vi "RH_Auto.vi"() -> ()   [LabVIEW 2012]
uses:
  <vilib>/ptbypt/NI_PtbyPt.lvlib
panel:
  out "Resistance [Ohm]":dbl=29.242166666666666 format="%#_6f"
  out "Lockin y (V)":dbl=2.45572e-05
  out "Lockin x (V)":dbl=0.000873212
  in  "On:Delta\nOff:Lock-in":bool
  in  "I for Lockin [A]":dbl=3e-05 format="%#_6e"
  out "Lockin Y (V)":dbl=2.41996e-05
  out "Lockin X (V)":dbl=0.000877265
  in  "Lockin SR830":refnum<visa-resource-name>="GPIB1::8::INSTR"
  in  "T-ramp off":bool
  in  "Main sorb T control":bool
  in  "Wait [min]":i32
  in  "LakeShore335":refnum<visa-resource-name>="COM4"
  in  "Temp control off":bool
  out "temp [K]":dbl=10.052
  out "Waiting T-stability":bool caption="stabilizing"
  in  "Set Initial Field":bool
  in  "Field [T]":dbl
  in  "Period [s]":dbl=0.5 caption="Delay Time (s)"
  in  "Measure R-T":bool
  in  "Save R-T":bool
  out "R-T":cluster{"X":dbl[], "Y":dbl[]}[](graph) caption="XY Graph"
  out "Rate [K/min]":dbl=-0.3439169609352251 format="%#_6f"
  in  "Reset":bool
  in  "Stop":bool
  in  "Pause off":bool
  in  "Compliance [V]":dbl=0.5 format="%#_6f"
  out "R-H":cluster{"X":dbl[], "Y":dbl[]}[](graph) caption="XY Graph"
  in  "Reset":bool
  in  "Folder":path=path "C:/User Data/Bart" caption="Filename"
  out "Filename Out":path=path "C:/User Data/Bart/CG013_RH_2_10.00K"
  in  "File name":string="CG013_RH_2"
  out "VTI [K]":dbl=9.9728
  out "VTI [K]":dbl=9.8121
  out "Sample Temp [K]":dbl=10.114
  out "Magnetic Field [T]":dbl=-2.97563
  out "Delta reading [Ohm]":dbl
  out "Delta Reading [Ohm]":dbl=11.9426813
  out "Sample Temp [K]":dbl=10.057
  in  "Abort Delta":bool
  in  "Arm Delta":bool
  in  "DELAY [sec]":dbl=0.002 format="%#_6e"
  in  "I-HIGH [A]":dbl=1e-06 format="%#_6e"
  in  "Measure R-H":bool
  in  "Rate [K/min]":dbl=0.5
  in  "Set Temp [K]":dbl=1.0
  in  "Set Temperature":bool
  out "Magnetic Field [T]":dbl=-2.94426
  in  "Rate [T/min]":dbl=0.5
  in  "Set Field [T]":dbl=3.0
  in  "Set Field":bool
  in  "Keithley":refnum<visa-resource-name>="GPIB1::20::INSTR"
  in  "Skip":bool
  in  "Wait T-stable [min]":i32=10
  in  "period (s)":dbl=0.5 min=0.0 max=1111.0 step=0.1
  in  "stop 2":bool caption="Pause"
  in  "Wait field stable [sec]":dbl=20.0
  in  "Magnet Power supply":refnum<visa-resource-name>="COM7"
  in  "Set Field [T]   Rate [T/min]":dbl[][](array[numeric])=[[0.0, 0.5], [3.0, 0.5], [0.0, 0.5], [-3.0, 0.5]]
  in  "Set Temp [K]  Rate [K/min]":dbl[][](array[numeric])=[[10.0, 3.0]]
  in  "LakeShore340":refnum<visa-resource-name>="GPIB1::4::INSTR"
  out "error out 3":errorcluster={"status"=FALSE, "code"=1073676294, "source"="VISA Read in RH_Auto.vi"}
  out "error out 2":errorcluster={"status"=FALSE, "code"=1073676294, "source"="VISA Read in RH_Auto.vi"}
  out "error out":errorcluster={"status"=FALSE, "code"=1073676294, "source"="VISA Read in RH_Auto.vi"}
  # "Manual control"
  # "R-H Auto Measurement"
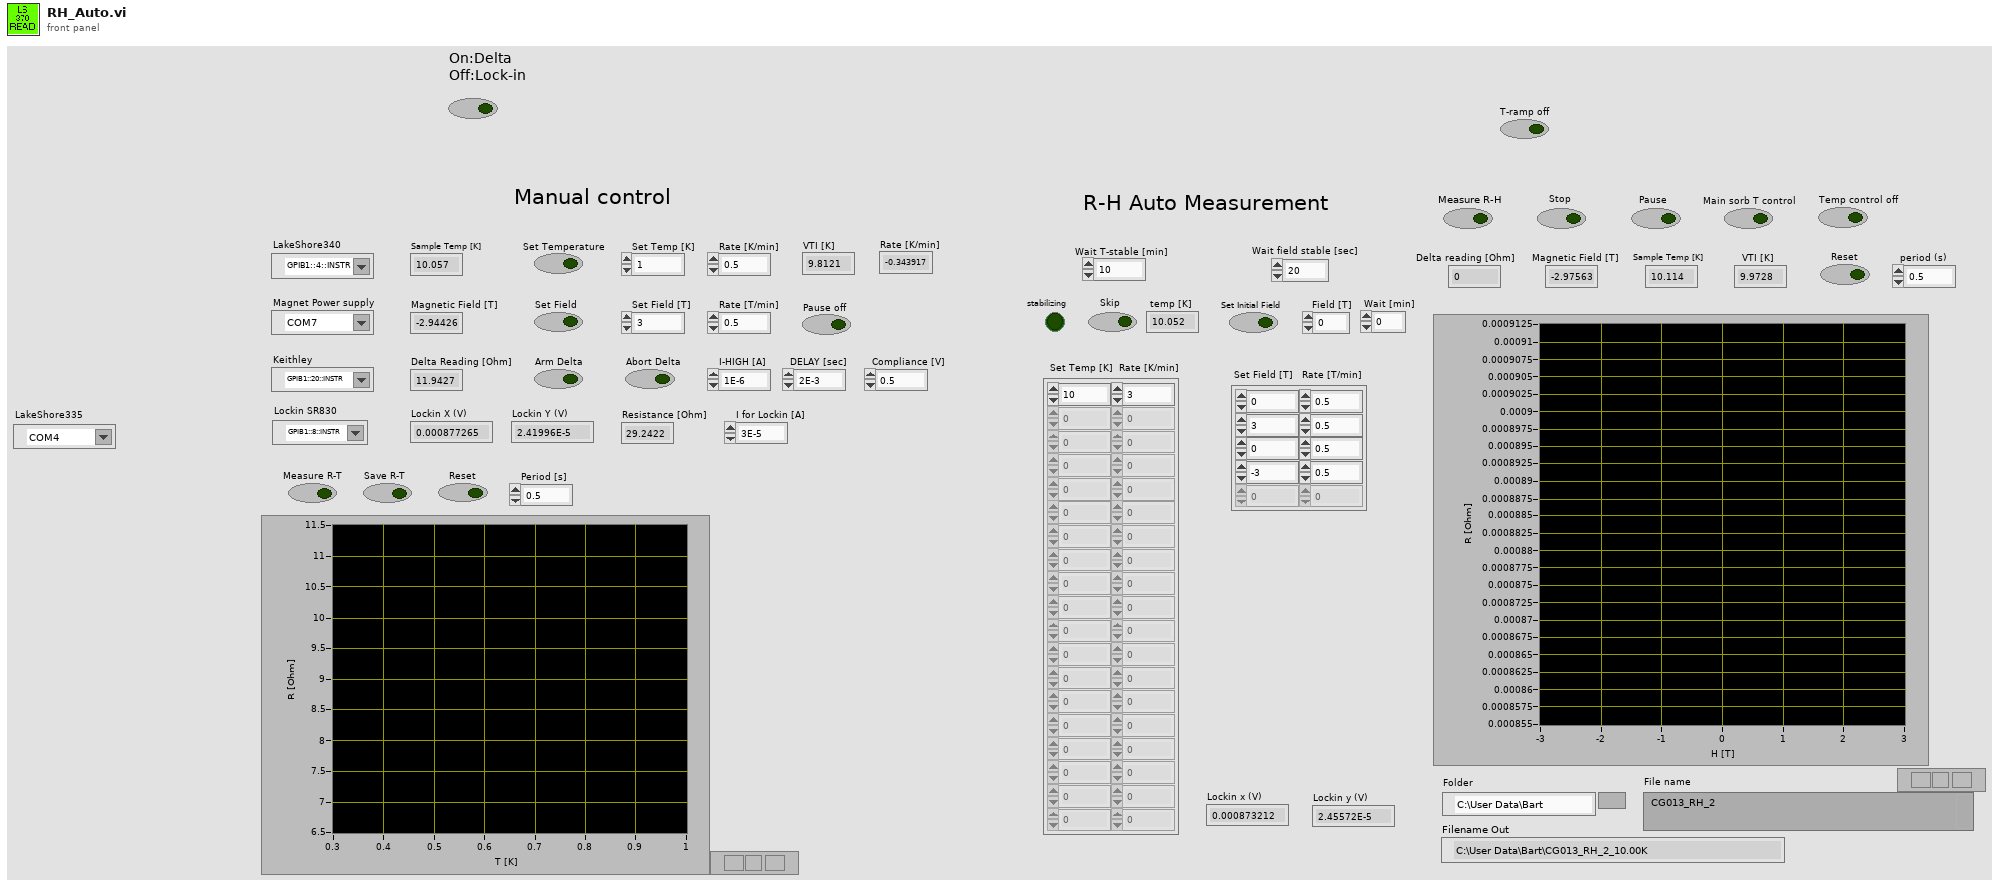
[diagram p1: front panel]
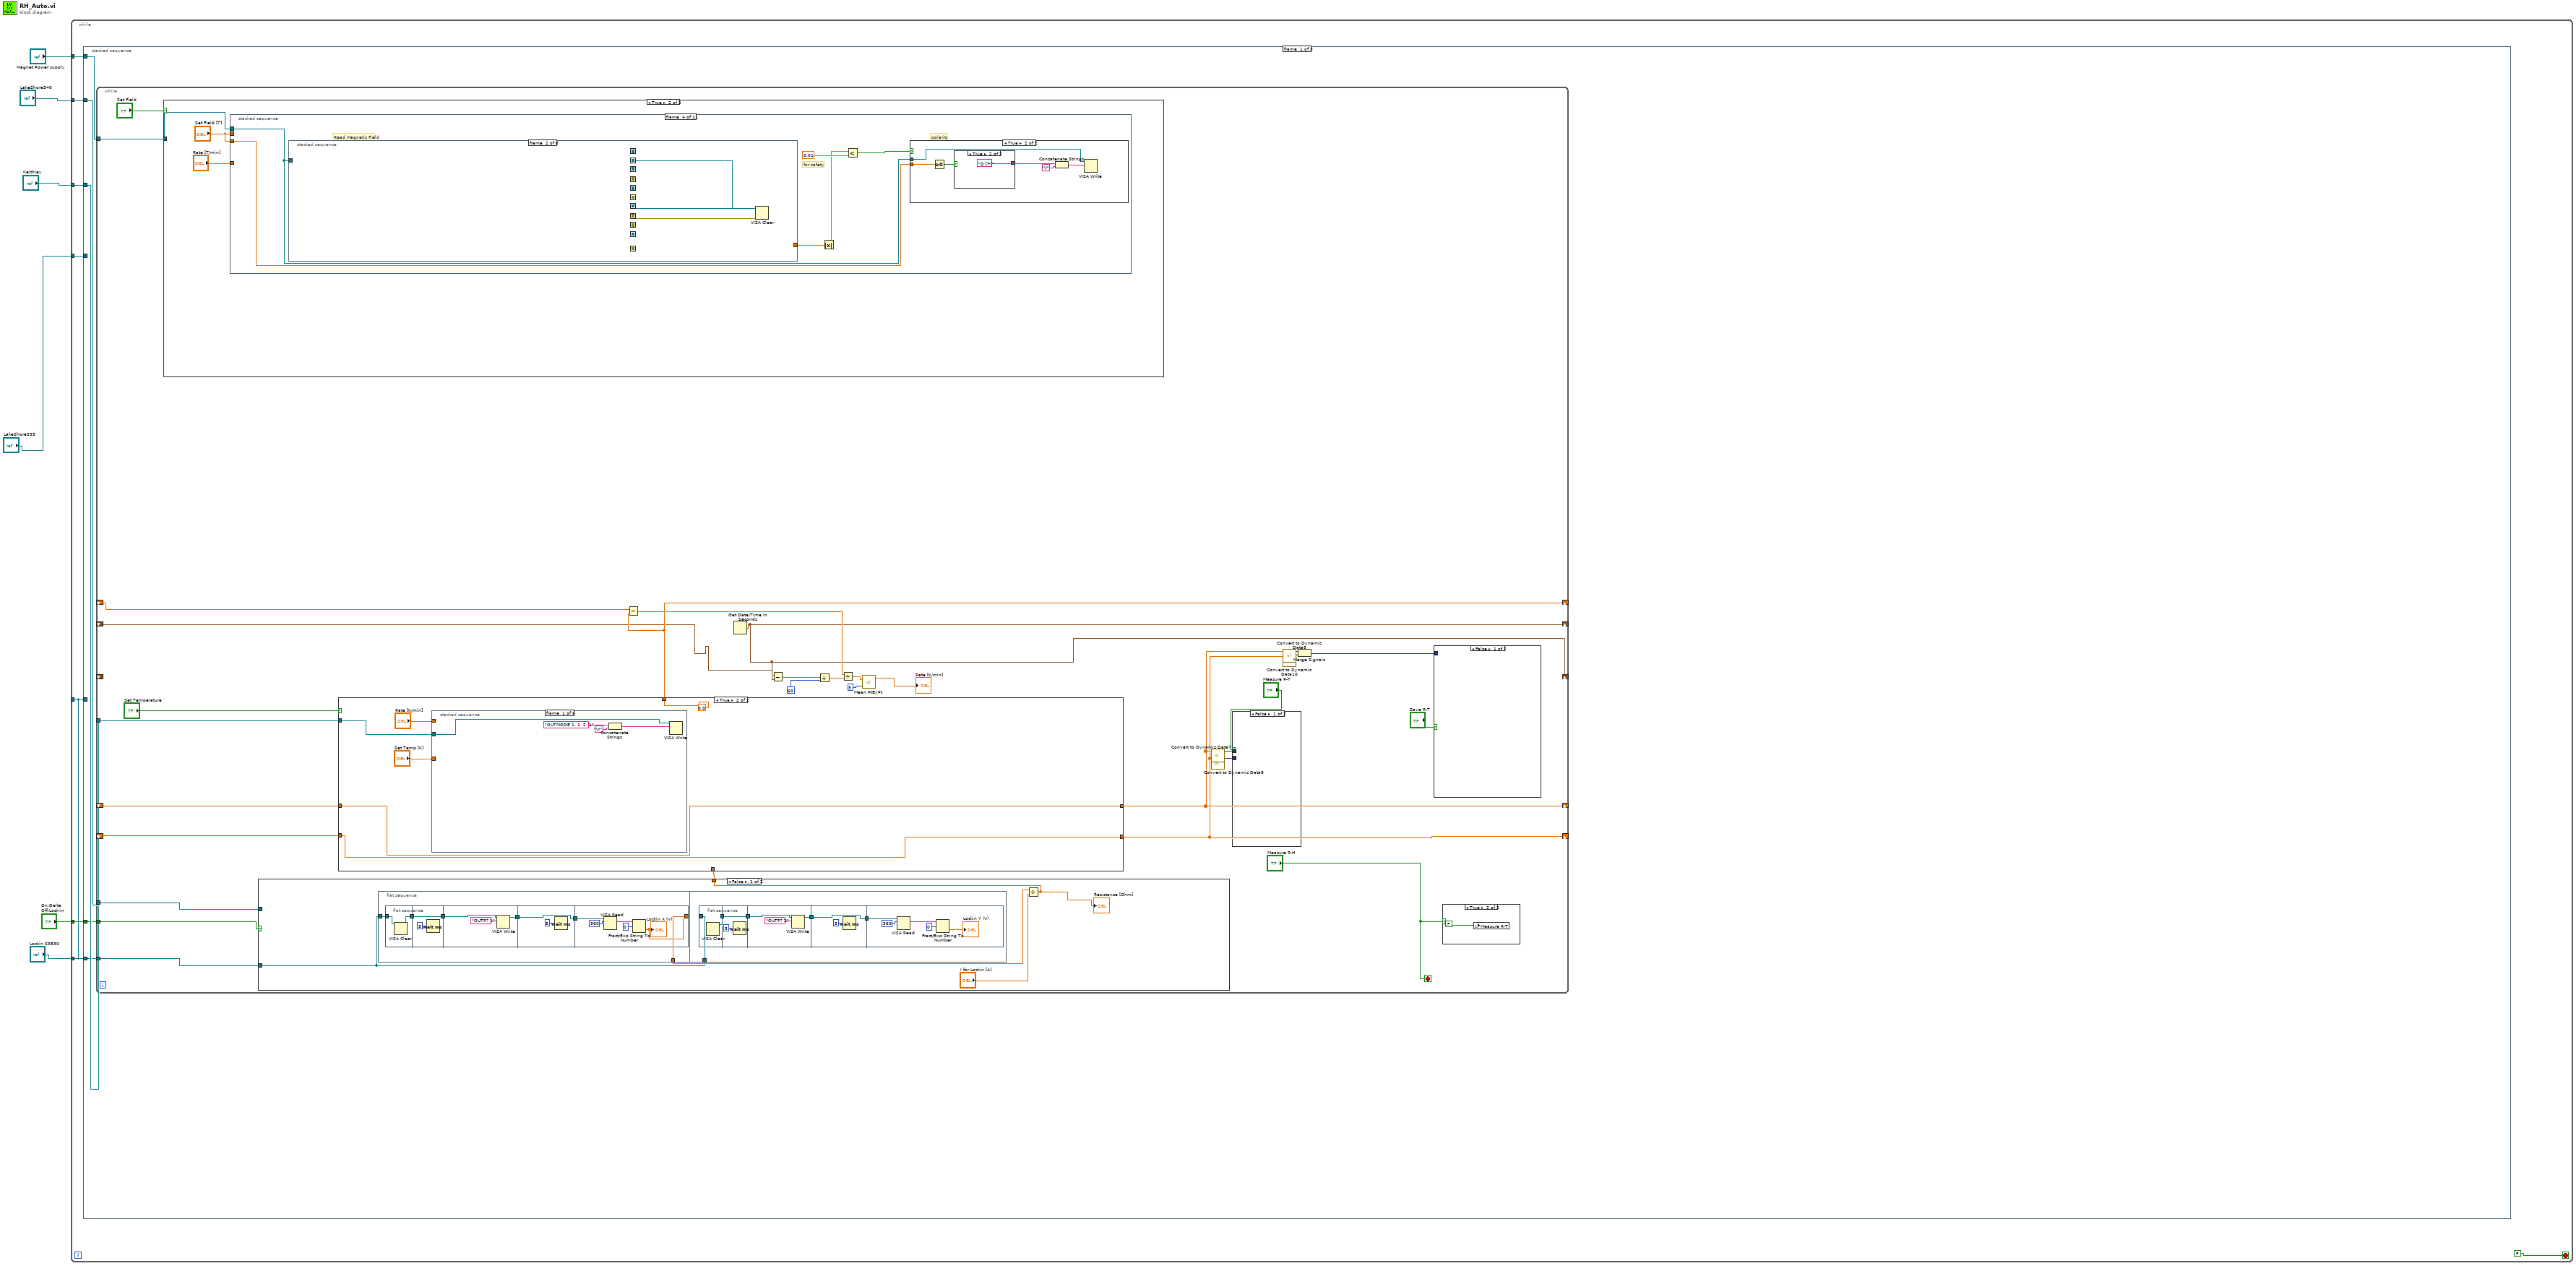
[diagram p0: block diagram]
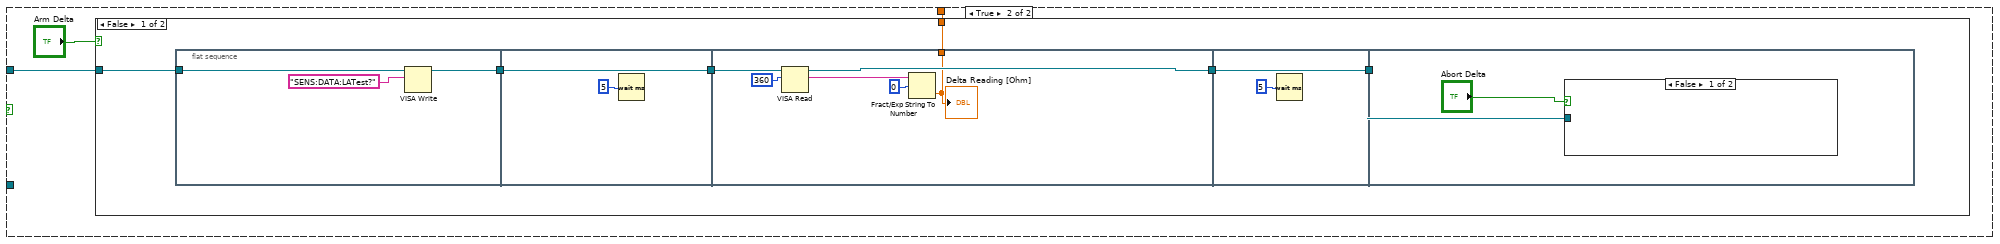
[diagram p2: hidden frame]
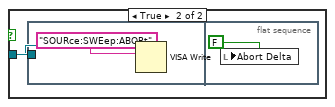
[diagram p3: hidden frame]
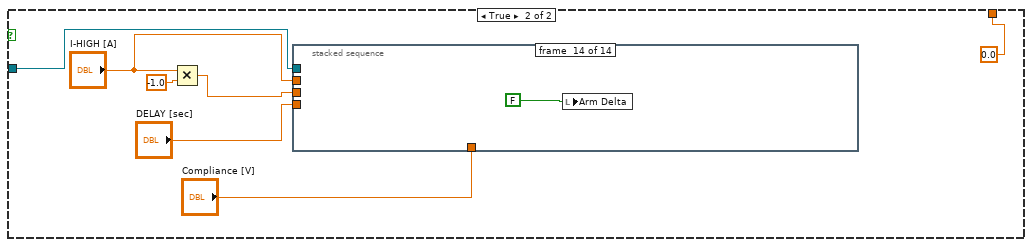
[diagram p4: hidden frame]
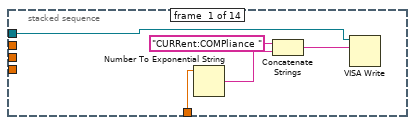
[diagram p5: hidden frame]
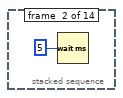
[diagram p6: hidden frame]
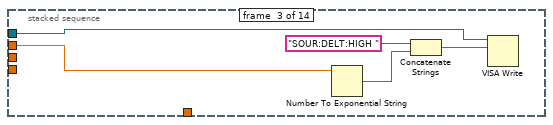
[diagram p7: hidden frame]
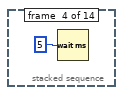
[diagram p8: hidden frame]
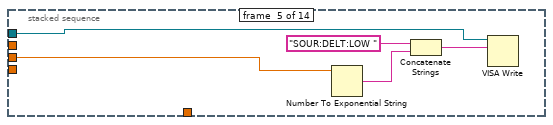
[diagram p9: hidden frame]
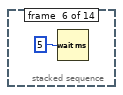
[diagram p10: hidden frame]
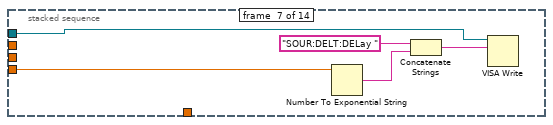
[diagram p11: hidden frame]
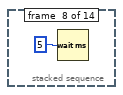
[diagram p12: hidden frame]
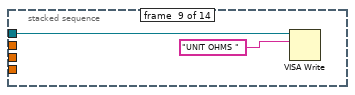
[diagram p13: hidden frame]
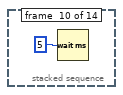
[diagram p14: hidden frame]
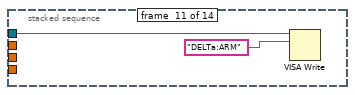
[diagram p15: hidden frame]
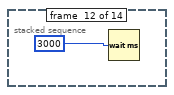
[diagram p16: hidden frame]
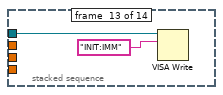
[diagram p17: hidden frame]
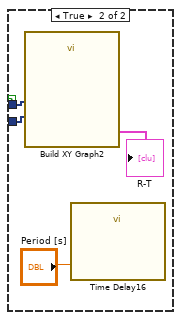
[diagram p19: hidden frame]
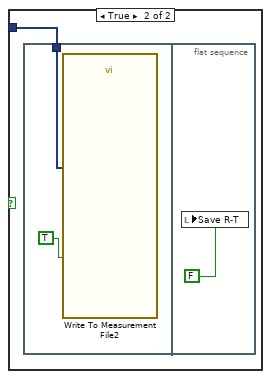
[diagram p20: hidden frame]
diagram:
  n1 = while {
    tunnel: "LakeShore340" -> [w13]
    tunnel: "Magnet Power supply" -> [w12]
    tunnel: "Keithley" -> [w11]
    tunnel: "LakeShore335" -> [w9]
    tunnel: "Lockin SR830" -> [w7]
    tunnel: "On:Delta\nOff:Lock-in" -> [w8]
    tunnel: [w7] -> _
    stop <- FALSE stop-if-true
    n2 = stacked-sequence {
      tunnel: w13 -> [w17 w408 _]
      tunnel: w12 -> [w18 w407 w999]
      tunnel: w11 -> [w16 w406 _]
      tunnel: w9 -> [_ w404 _]
      tunnel: w7 -> [w15 _ _]
      tunnel: w8 -> [w14 w403 _]
      tunnel: w7 -> [_ w402 _]
      frame #0 {
        n3 = while {
          tunnel: w18 -> [w45]
          tunnel: w17 -> [w47]
          tunnel: w16 -> [w46]
          shift-right: [w33] -> _
          shift-left: _ -> [w28]
          shift-right: [w31] -> _
          shift-left: _ -> [w43]
          shift-right: [w25] -> _
          shift-left: _ -> [_]
          shift-right: [w41] -> _
          shift-left: _ -> [w42]
          shift-right: [w25] -> _
          shift-left: _ -> [w24]
          tunnel: w15 -> [w20]
          tunnel: w14 -> [w19]
          stop <- "Measure R-H" stop-if-true
          n4 = case shown="True" "Set Field" {
            tunnel: w45 -> [w237 w307]
            frame False {
              n5 = stacked-sequence {
                seq-local: [w238 _ _ _ _ _ _ _] -> [_ w241 _ _ _ _ _ _]
                seq-local: [_ w239 _ _ _ _ _ _] -> [_ _ w245 _ _ _ _ _]
                seq-local: [_ w240 _ _ _ _ _ _] -> [_ _ w242 _ _ _ _ _]
                seq-local: [_ _ w244 _ _ _ _ _] -> [_ _ _ w285 _ _ _ _]
                seq-local: [_ _ w243 _ _ _ _ _] -> [_ _ _ w284 _ _ _ _]
                seq-local: [_ _ _ w287 _ _ _ _] -> [_ _ _ _ w290 _ _ _]
                seq-local: [_ _ _ w286 _ _ _ _] -> [_ _ _ _ w291 _ _ _]
                seq-local: [_ _ _ _ w290 _ _ _] -> [_ _ _ _ _ w302 _ _]
                seq-local: [_ _ _ _ w291 _ _ _] -> [_ _ _ _ _ w300 _ _]
                seq-local: [_ _ _ _ _ w301 _ _] -> [_ _ _ _ _ _ _ w306]
                seq-local: [_ _ _ _ _ w299 _ _] -> [_ _ _ _ _ _ _ w305]
                tunnel: w237 -> [w238 _ _ _ _ _ _ _]
                tunnel: [_ _ _ _ _ w292 _ _] -> w236
                frame #0 {
                }
                frame #1 {
                  n6 = VISA Clear(VISA resource name=w241) -> (VISA resource name out=w239:refnum<visa-resource-name>, error out=w240:errorcluster)  [unwired: 1 in]
                }
                frame #2 {
                  n7 = flat-sequence {
                    tunnel: w245 -> [w249]
                    tunnel: [w248] -> w244
                    tunnel: [w247] -> w243
                    tunnel: w242 -> [w246]
                    frame #0 {
                      n8 = call "Time Delay8"() -> ()  [unwired: 11 in, 1 out]
                    }
                    frame #1 {
                      n9 = case shown="False" "Pause off" {
                        tunnel: w249 -> [w252 w264]
                        tunnel: [w252 w253] -> w248
                        tunnel: [w251 w256] -> w247
                        tunnel: w246 -> [w251 w259]
                        frame False {
                        }
                        frame True {
                          n10 = flat-sequence {
                            tunnel: w264 -> [w268]
                            tunnel: [w267] -> w262
                            tunnel: [w266] -> w260
                            tunnel: w259 -> [w265]
                            tunnel: [w273] -> w263
                            tunnel: w262 -> [w273]
                            tunnel: [w272] -> w261
                            tunnel: w260 -> [w272]
                            tunnel: w263 -> [w275]
                            tunnel: w261 -> [_]
                            tunnel: [w275] -> w258
                            tunnel: [w274] -> w254
                            tunnel: w258 -> [w277]
                            tunnel: [w277] -> w257
                            tunnel: [w276] -> w255
                            tunnel: w254 -> [w276]
                            tunnel: [w281] -> w253
                            tunnel: w257 -> [w280]
                            tunnel: [w279] -> w256
                            tunnel: w255 -> [w278]
                            frame #0 {
                              n11 = Concatenate Strings("P 0" ("Command"), "\r") -> (w270:string)
                              n12 = VISA Write(VISA resource name=w268, write buffer=w270, error in (no error)=w265) -> (VISA resource name out=w267:refnum<visa-resource-name>, error out=w266:errorcluster)  [unwired: 1 out]
                            }
                            frame #1 {
                              n13 = call "Time Delay14"() -> ()  [unwired: 11 in, 1 out]
                            }
                            frame #2 {
                              n14 = VISA Close(VISA resource name=w275) -> (error out=w274:errorcluster)  [unwired: 1 in]
                            }
                            frame #3 {
                              n15 = call "Time Delay15"() -> ()  [unwired: 11 in, 1 out]
                            }
                            frame #4 {
                              n16 = VISA Clear(VISA resource name=w280, error in (no error)=w278) -> (VISA resource name out=w281:refnum<visa-resource-name>, error out=w279:errorcluster)
                            }
                            frame #5 {
                              n17 = local write "Pause off"(FALSE) -> ()
                            }
                          }
                        }
                      }
                    }
                  }
                }
                frame #3 {
                  n18 = Concatenate Strings("G O" ("Command"), "\r") -> (w288:string)
                  n19 = VISA Write(VISA resource name=w285, write buffer=w288, error in (no error)=w284) -> (VISA resource name out=w287:refnum<visa-resource-name>, error out=w286:errorcluster)  [unwired: 1 out]
                }
                frame #4 {
                  n20 = call "Time Delay9"() -> ()  [unwired: 11 in, 1 out]
                }
                frame #5 {
                  n21 = VISA Read(VISA resource name=w302, byte count=u32 30, error in (no error)=w300) -> (VISA resource name out=w301:refnum<visa-resource-name>, read buffer=w296:string, error out=w299:errorcluster)  [unwired: 1 out]
                  n22 = Match Pattern(string=w296, regular expression="OUTPUT:") -> (after substring=w294:string)  [unwired: 1 in, 3 out]
                  n23 = Match Pattern(string=w294, regular expression=" TESLA") -> (before substring=w293:string)  [unwired: 1 in, 3 out]
                  n24 = Fract/Exp String To Number(string=w293, offset=0) -> (number=w292:dbl)  [unwired: 2 in, 1 out]
                }
                frame #6 {
                  n25 = call "Time Delay10"() -> ()  [unwired: 11 in, 1 out]
                }
                frame #7 {
                  n26 = VISA Close(VISA resource name=w306, error in (no error)=w305) -> (error out=→"error out":errorcluster)
                }
              }
              "Magnetic Field [T]" <- w236
            }
            frame True {
              n27 = stacked-sequence {
                tunnel: w307 -> [w310 _ _ w329 _ w374 _ w392 _ w397 _]
                tunnel: "Set Field [T]" -> [_ w312 _ _ _ _ _ _ _ _ _]
                tunnel: "Rate [T/min]" -> [_ w311 _ _ _ _ _ w382 _ _ _]
                tunnel: "Set Field [T]" -> [_ _ _ w328 _ w372 _ _ _ _ _]
                frame #0 {
                  n28 = VISA Clear(VISA resource name=w310) -> ()  [unwired: 1 in, 2 out]
                }
                frame #1 {
                  n29 = Greater?(x=w312, y=10) -> (0:w313:bool)
                  n30 = Less?(x=w312, y=-10) -> (x < y?=w318:bool)
                  n31 = Greater?(x=w311, y=0.6) -> (0:w322:bool)
                  n32 = Less?(x=w311, y=-0.6) -> (x < y?=w321:bool)
                  n33 = Or(x=w313, y=w318) -> (x .or. y?=w324:bool)
                  n34 = Or(x=w322, y=w321) -> (x .or. y?=w323:bool)
                  n35 = call "Display Message to User6"("Enable"=w324) -> ("OK"=w325:bool)  [unwired: 9 in, 1 out]
                  n36 = call "Display Message to User5"("Enable"=w323) -> ("OK"=w314:bool)  [unwired: 9 in, 1 out]
                  n37 = Or(x=w325, y=w314) -> (x .or. y?=w315:bool)
                  n38 = Stop(stop? (T)=w315) -> ()
                }
                frame #2 {
                  n39 = Wait (ms)(milliseconds to wait=500) -> ()  [unwired: 1 out]
                }
                frame #3 {
                  # "Read Magnetic Field"
                  # "for safety"
                  # "polarity"
                  n40 = stacked-sequence {
                    seq-local: [w333 _ _ _ _ _ _ _] -> [_ w336 _ _ _ _ _ _]
                    seq-local: [_ w334 _ _ _ _ _ _] -> [_ _ w338 _ _ _ _ _]
                    seq-local: [_ w335 _ _ _ _ _ _] -> [_ _ w337 _ _ _ _ _]
                    seq-local: [_ _ w338 _ _ _ _ _] -> [_ _ _ w341 _ _ _ _]
                    seq-local: [_ _ w337 _ _ _ _ _] -> [_ _ _ w340 _ _ _ _]
                    seq-local: [_ _ _ w343 _ _ _ _] -> [_ _ _ _ w346 _ _ _]
                    seq-local: [_ _ _ w342 _ _ _ _] -> [_ _ _ _ w347 _ _ _]
                    seq-local: [_ _ _ _ w346 _ _ _] -> [_ _ _ _ _ w358 _ _]
                    seq-local: [_ _ _ _ w347 _ _ _] -> [_ _ _ _ _ w356 _ _]
                    seq-local: [_ _ _ _ _ w357 _ _] -> [_ _ _ _ _ _ _ w362]
                    seq-local: [_ _ _ _ _ w355 _ _] -> [_ _ _ _ _ _ _ w361]
                    tunnel: w329 -> [w333 _ _ _ _ _ _ _]
                    tunnel: [_ _ _ _ _ w348 _ _] -> w330
                    frame #0 {
                    }
                    frame #1 {
                      n41 = VISA Clear(VISA resource name=w336) -> (VISA resource name out=w334:refnum<visa-resource-name>, error out=w335:errorcluster)  [unwired: 1 in]
                    }
                    frame #2 {
                      n42 = call "Time Delay6"() -> ()  [unwired: 11 in, 1 out]
                    }
                    frame #3 {
                      n43 = Concatenate Strings("G O" ("Command"), "\r") -> (w344:string)
                      n44 = VISA Write(VISA resource name=w341, write buffer=w344, error in (no error)=w340) -> (VISA resource name out=w343:refnum<visa-resource-name>, error out=w342:errorcluster)  [unwired: 1 out]
                    }
                    frame #4 {
                      n45 = call "Time Delay7"() -> ()  [unwired: 11 in, 1 out]
                    }
                    frame #5 {
                      n46 = VISA Read(VISA resource name=w358, byte count=u32 30, error in (no error)=w356) -> (VISA resource name out=w357:refnum<visa-resource-name>, read buffer=w352:string, error out=w355:errorcluster)  [unwired: 1 out]
                      n47 = Match Pattern(string=w352, regular expression="OUTPUT:") -> (after substring=w350:string)  [unwired: 1 in, 3 out]
                      n48 = Match Pattern(string=w350, regular expression=" TESLA") -> (before substring=w349:string)  [unwired: 1 in, 3 out]
                      n49 = Fract/Exp String To Number(string=w349, offset=0) -> (number=w348:dbl)  [unwired: 2 in, 1 out]
                    }
                    frame #6 {
                      n50 = call "Time Delay11"() -> ()  [unwired: 11 in, 1 out]
                    }
                    frame #7 {
                      n51 = VISA Close(VISA resource name=w362, error in (no error)=w361) -> (error out=→"error out 2":errorcluster)
                    }
                  }
                  n52 = Absolute Value(x=w330) -> (abs(x)=w331:dbl)
                  n53 = Less?(x=w331, y=0.01) -> (x < y?=w327:bool)
                  n54 = case shown="True" w327 {
                    tunnel: w329 -> [_ w365]
                    tunnel: w328 -> [_ w363]
                    frame False {
                    }
                    frame True {
                      n55 = Greater Or Equal To 0?(x=w363) -> (x >= 0?=w364:bool)
                      n56 = case shown="True" w364 {
                        tunnel: ["D [-]" ("data") "D [+]" ("data")] -> w366
                        frame False {
                        }
                        frame True {
                        }
                      }
                      n57 = Concatenate Strings(w366, "\r") -> (w368:string)
                      n58 = VISA Write(VISA resource name=w365, write buffer=w368) -> ()  [unwired: 1 in, 3 out]
                    }
                  }
                }
                frame #4 {
                  n59 = Wait (ms)(milliseconds to wait=500) -> ()  [unwired: 1 out]
                }
                frame #5 {
                  # "set set field"
                  n60 = Number To Fractional String(number=w372, width (-)=i16 6, precision (6)=i16 3) -> (F-format string=w377:string)  [unwired: 1 in]
                  n61 = Concatenate Strings("S [%][MID] " ("string"), w377) -> (w373:string)
                  n62 = Concatenate Strings(w373, "\r") -> (w376:string)
                  n63 = VISA Write(VISA resource name=w374, write buffer=w376) -> ()  [unwired: 1 in, 3 out]
                }
                frame #6 {
                  n64 = Wait (ms)(milliseconds to wait=500) -> ()  [unwired: 1 out]
                }
                frame #7 {
                  # "set rate"
                  n65 = Divide(x=w382, y=60.0) -> (x/y=w387:dbl)
                  n66 = Divide(x=w387, y=0.09797) -> (x/y=w385:dbl)
                  n67 = Number To Fractional String(number=w385, width (-)=i16 6, precision (6)=i16 3) -> (F-format string=w390:string)  [unwired: 1 in]
                  n68 = Concatenate Strings("S R " ("string"), w390) -> (w389:string)
                  n69 = Concatenate Strings(w389, "\r") -> (w394:string)
                  n70 = VISA Write(VISA resource name=w392, write buffer=w394) -> ()  [unwired: 1 in, 3 out]
                }
                frame #8 {
                  n71 = Wait (ms)(milliseconds to wait=500) -> ()  [unwired: 1 out]
                }
                frame #9 {
                  # "Go to set field"
                  n72 = Concatenate Strings("R [%][MID]" ("data"), "\r") -> (w399:string)
                  n73 = VISA Write(VISA resource name=w397, write buffer=w399) -> ()  [unwired: 1 in, 3 out]
                }
                frame #10 {
                  n74 = local write "Set Field"(FALSE) -> ()
                  n75 = Wait (ms)(milliseconds to wait=500) -> ()  [unwired: 1 out]
                }
              }
            }
          }
          n76 = case shown="False" w19 {
            tunnel: w46 -> [_ w95]
            tunnel: [w50 w93] -> w44
            tunnel: w20 -> [w51 _]
            frame False {
              n77 = flat-sequence {
                tunnel: [w57] -> w52
                tunnel: w51 -> [w56]
                tunnel: w51 -> [w76]
                frame #0 {
                  n78 = flat-sequence {
                    tunnel: w56 -> [w61]
                    tunnel: [w60] -> w54
                    tunnel: [w63] -> w55
                    tunnel: w54 -> [w63]
                    tunnel: [w64] -> w59
                    tunnel: w55 -> [w66]
                    tunnel: [w67] -> w58
                    tunnel: w59 -> [w67]
                    tunnel: w58 -> [w71]
                    tunnel: [w69] -> w57
                    frame #0 {
                      n79 = VISA Clear(VISA resource name=w61) -> (VISA resource name out=w60:refnum<visa-resource-name>)  [unwired: 1 in, 1 out]
                    }
                    frame #1 {
                      n80 = Wait (ms)(milliseconds to wait=5) -> ()  [unwired: 1 out]
                    }
                    frame #2 {
                      n81 = VISA Write(VISA resource name=w66, write buffer="OUTP? 1" ("write buffer 2")) -> (VISA resource name out=w64:refnum<visa-resource-name>)  [unwired: 1 in, 2 out]
                    }
                    frame #3 {
                      n82 = Wait (ms)(milliseconds to wait=5) -> ()  [unwired: 1 out]
                    }
                    frame #4 {
                      n83 = VISA Read(VISA resource name=w71, byte count=u32 360) -> (read buffer=w70:string)  [unwired: 1 in, 3 out]
                      n84 = Fract/Exp String To Number(string=w70, offset=0) -> (number=w69:dbl)  [unwired: 3 out]
                      "Lockin X (V)" <- w69
                    }
                  }
                }
                frame #1 {
                  n85 = flat-sequence {
                    tunnel: w76 -> [w80]
                    tunnel: [w79] -> w74
                    tunnel: [w82] -> w75
                    tunnel: w74 -> [w82]
                    tunnel: [w83] -> w78
                    tunnel: w75 -> [w85]
                    tunnel: [w86] -> w77
                    tunnel: w78 -> [w86]
                    tunnel: w77 -> [w90]
                    frame #0 {
                      n86 = VISA Clear(VISA resource name=w80) -> (VISA resource name out=w79:refnum<visa-resource-name>)  [unwired: 1 in, 1 out]
                    }
                    frame #1 {
                      n87 = Wait (ms)(milliseconds to wait=5) -> ()  [unwired: 1 out]
                    }
                    frame #2 {
                      n88 = VISA Write(VISA resource name=w85, write buffer="OUTP? 2" ("write buffer 2")) -> (VISA resource name out=w83:refnum<visa-resource-name>)  [unwired: 1 in, 2 out]
                    }
                    frame #3 {
                      n89 = Wait (ms)(milliseconds to wait=5) -> ()  [unwired: 1 out]
                    }
                    frame #4 {
                      n90 = VISA Read(VISA resource name=w90, byte count=u32 360) -> (read buffer=w89:string)  [unwired: 1 in, 3 out]
                      n91 = Fract/Exp String To Number(string=w89, offset=0) -> (number=→"Lockin Y (V)":dbl)  [unwired: 3 out]
                    }
                  }
                }
              }
              n92 = Divide(x=w52, y="I for Lockin [A]") -> (x/y=w50:dbl)
              "Resistance [Ohm]" <- w50
            }
            frame True {
              n93 = case shown="False" "Arm Delta" {
                tunnel: w95 -> [w101 w125]
                tunnel: [w96 0.0] -> w93
                frame False {
                  n94 = flat-sequence {
                    tunnel: w101 -> [w104]
                    tunnel: [w102] -> w99
                    tunnel: [w105] -> w100
                    tunnel: w99 -> [w105]
                    tunnel: w100 -> [w109]
                    tunnel: [w108] -> w97
                    tunnel: [w107] -> w96
                    tunnel: [w113] -> w98
                    tunnel: w97 -> [w113]
                    tunnel: w98 -> [w115]
                    frame #0 {
                      n95 = VISA Write(VISA resource name=w104, write buffer="SENS:DATA:LATest?" ("write buffer 2")) -> (VISA resource name out=w102:refnum<visa-resource-name>)  [unwired: 1 in, 2 out]
                    }
                    frame #1 {
                      n96 = Wait (ms)(milliseconds to wait=5) -> ()  [unwired: 1 out]
                    }
                    frame #2 {
                      n97 = VISA Read(VISA resource name=w109, byte count=u32 360) -> (VISA resource name out=w108:refnum<visa-resource-name>, read buffer=w111:string)  [unwired: 1 in, 2 out]
                      n98 = Fract/Exp String To Number(string=w111, offset=0) -> (number=w107:dbl)  [unwired: 3 out]
                      "Delta Reading [Ohm]" <- w107
                    }
                    frame #3 {
                      n99 = Wait (ms)(milliseconds to wait=5) -> ()  [unwired: 1 out]
                    }
                    frame #4 {
                      n100 = case shown="False" "Abort Delta" {
                        tunnel: w115 -> [_ w117]
                        frame False {
                        }
                        frame True {
                          n101 = flat-sequence {
                            tunnel: w117 -> [w119]
                            frame #0 {
                              n102 = VISA Write(VISA resource name=w119, write buffer="SOURce:SWEep:ABORt") -> ()  [unwired: 1 in, 3 out]
                            }
                            frame #1 {
                              n103 = local write "Abort Delta"(FALSE) -> ()
                            }
                          }
                        }
                      }
                    }
                  }
                }
                frame True {
                  n104 = Multiply(x="I-HIGH [A]", y=-1.0) -> (x*y=w124:dbl)
                  n105 = stacked-sequence {
                    tunnel: "I-HIGH [A]" -> [_ _ w136 _ _ _ _ _ _ _ _ _ _ _]
                    tunnel: w125 -> [w129 _ w134 _ w141 _ w147 _ w152 _ w155 _ w158 _]
                    tunnel: w124 -> [_ _ _ _ w140 _ _ _ _ _ _ _ _ _]
                    tunnel: "DELAY [sec]" -> [_ _ _ _ _ _ w146 _ _ _ _ _ _ _]
                    tunnel: "Compliance [V]" -> [w128 _ _ _ _ _ _ _ _ _ _ _ _ _]
                    frame #0 {
                      n106 = Number To Exponential String(number=w128) -> (E-format string=w131:string)  [unwired: 3 in]
                      n107 = Concatenate Strings("CURRent:COMPliance ", w131) -> (w130:string)
                      n108 = VISA Write(VISA resource name=w129, write buffer=w130) -> ()  [unwired: 1 in, 3 out]
                    }
                    frame #1 {
                      n109 = Wait (ms)(milliseconds to wait=5) -> ()  [unwired: 1 out]
                    }
                    frame #2 {
                      n110 = Number To Exponential String(number=w136) -> (E-format string=w137:string)  [unwired: 3 in]
                      n111 = Concatenate Strings("SOUR:DELT:HIGH ", w137) -> (w135:string)
                      n112 = VISA Write(VISA resource name=w134, write buffer=w135) -> ()  [unwired: 1 in, 3 out]
                    }
                    frame #3 {
                      n113 = Wait (ms)(milliseconds to wait=5) -> ()  [unwired: 1 out]
                    }
                    frame #4 {
                      n114 = Number To Exponential String(number=w140) -> (E-format string=w143:string)  [unwired: 3 in]
                      n115 = Concatenate Strings("SOUR:DELT:LOW ", w143) -> (w142:string)
                      n116 = VISA Write(VISA resource name=w141, write buffer=w142) -> ()  [unwired: 1 in, 3 out]
                    }
                    frame #5 {
                      n117 = Wait (ms)(milliseconds to wait=5) -> ()  [unwired: 1 out]
                    }
                    frame #6 {
                      n118 = Number To Exponential String(number=w146) -> (E-format string=w149:string)  [unwired: 3 in]
                      n119 = Concatenate Strings("SOUR:DELT:DELay ", w149) -> (w148:string)
                      n120 = VISA Write(VISA resource name=w147, write buffer=w148) -> ()  [unwired: 1 in, 3 out]
                    }
                    frame #7 {
                      n121 = Wait (ms)(milliseconds to wait=5) -> ()  [unwired: 1 out]
                    }
                    frame #8 {
                      n122 = VISA Write(VISA resource name=w152, write buffer="UNIT OHMS ") -> ()  [unwired: 1 in, 3 out]
                    }
                    frame #9 {
                      n123 = Wait (ms)(milliseconds to wait=5) -> ()  [unwired: 1 out]
                    }
                    frame #10 {
                      n124 = VISA Write(VISA resource name=w155, write buffer="DELTa:ARM") -> ()  [unwired: 1 in, 3 out]
                    }
                    frame #11 {
                      n125 = Wait (ms)(milliseconds to wait=3000) -> ()  [unwired: 1 out]
                    }
                    frame #12 {
                      n126 = VISA Write(VISA resource name=w158, write buffer="INIT:IMM") -> ()  [unwired: 1 in, 3 out]
                    }
                    frame #13 {
                      n127 = local write "Arm Delta"(FALSE) -> ()
                    }
                  }
                }
              }
            }
          }
          n128 = case shown="True" "Set Temperature" {
            tunnel: w47 -> [w180 w216]
            tunnel: [w175 w213] -> w33
            tunnel: w28 -> [w176 w213]
            tunnel: w44 -> [w174 _]
            tunnel: [w173 w212] -> w31
            tunnel: w43 -> [w172 w212]
            tunnel: [w170 0.0] -> w41
            frame False {
              n129 = flat-sequence {
                tunnel: w180 -> [w194]
                tunnel: [w193] -> w178
                tunnel: [w192] -> w177
                tunnel: [w192] -> w170
                tunnel: [w201] -> w179
                tunnel: w178 -> [w201]
                tunnel: w179 -> [w203]
                frame #0 {
                  n130 = Concatenate Strings("KRDG?B" ("write buffer"), "\n") -> (w199:string)
                  n131 = VISA Write(VISA resource name=w194, write buffer=w199) -> (VISA resource name out=w197:refnum<visa-resource-name>)  [unwired: 1 in, 2 out]
                  n132 = VISA Read(VISA resource name=w197, byte count=u32 100) -> (VISA resource name out=w193:refnum<visa-resource-name>, read buffer=w195:string)  [unwired: 1 in, 2 out]
                  n133 = Fract/Exp String To Number(string=w195) -> (number=w192:dbl)  [unwired: 3 in, 1 out]
                  "Sample Temp [K]" <- w192
                }
                frame #1 {
                  n134 = Wait (ms)(milliseconds to wait=5) -> ()  [unwired: 1 out]
                }
                frame #2 {
                  n135 = Concatenate Strings("KRDG?A" ("write buffer"), "\n") -> (w209:string)
                  n136 = VISA Write(VISA resource name=w203, write buffer=w209) -> (VISA resource name out=w207:refnum<visa-resource-name>)  [unwired: 1 in, 2 out]
                  n137 = VISA Read(VISA resource name=w207, byte count=u32 100) -> (read buffer=w205:string)  [unwired: 1 in, 3 out]
                  n138 = Fract/Exp String To Number(string=w205) -> (number=→"VTI [K]":dbl)  [unwired: 3 in, 1 out]
                }
              }
              n139 = case shown="False" "Reset" {
                tunnel: w177 -> [w186 _]
                tunnel: w176 -> [w185 _]
                tunnel: [w184 w188] -> w175
                tunnel: w174 -> [w183 _]
                tunnel: [w182 w187] -> w173
                tunnel: w172 -> [w181 _]
                frame False {
                  n140 = Build Array (concatenate)(w185, w186) -> (w184:dbl[])
                  n141 = Build Array (concatenate)(w181, w183) -> (w182:dbl[])
                }
                frame True {
                  n142 = stacked-sequence {
                    tunnel: [dbl[] [] _] -> w188
                    tunnel: [dbl[] [] _] -> w187
                    frame #0 {
                    }
                    frame #1 {
                      n143 = local write "Reset"(FALSE) -> ()
                    }
                  }
                }
              }
            }
            frame True {
              n144 = stacked-sequence {
                tunnel: w216 -> [w217 _ w224 _ w231 _]
                tunnel: "Set Temp [K]" -> [_ _ _ _ w229 _]
                tunnel: "Rate [K/min]" -> [_ _ w223 _ _ _]
                frame #0 {
                  n145 = Concatenate Strings("OUTMODE 1, 1, 2, 1" ("write buffer"), "\n") -> (w218:string)
                  n146 = VISA Write(VISA resource name=w217, write buffer=w218) -> ()  [unwired: 1 in, 3 out]
                }
                frame #1 {
                  n147 = Wait (ms)(milliseconds to wait=u32 50) -> ()  [unwired: 1 out]
                }
                frame #2 {
                  n148 = Number To Fractional String(number=w223) -> (F-format string=w222:string)  [unwired: 3 in]
                  n149 = Concatenate Strings("RAMP 1, 1," ("write buffer"), w222, "\n") -> (w226:string)
                  n150 = VISA Write(VISA resource name=w224, write buffer=w226) -> ()  [unwired: 1 in, 3 out]
                }
                frame #3 {
                  n151 = Wait (ms)(milliseconds to wait=u32 50) -> ()  [unwired: 1 out]
                }
                frame #4 {
                  n152 = Number To Fractional String(number=w229) -> (F-format string=w230:string)  [unwired: 3 in]
                  n153 = Concatenate Strings("SETP 1," ("write buffer"), w230, "\n") -> (w233:string)
                  n154 = VISA Write(VISA resource name=w231, write buffer=w233) -> ()  [unwired: 1 in, 3 out]
                }
                frame #5 {
                  n155 = local write "Set Temperature"(FALSE) -> ()
                }
              }
            }
          }
          n156 = Subtract(x=w42, y=w41) -> (x-y=w37:dbl)
          n157 = Get Date/Time In Seconds() -> (seconds since 1Jan1904=w25:timestamp)
          n158 = Subtract(x=w24, y=w25) -> (x-y=w40:dbl)
          n159 = Divide(x=w40, y=60) -> (x/y=w38:dbl)
          n160 = Divide(x=w37, y=w38) -> (x/y=w22:dbl)
          n161 = call <vilib>:"Mean PtByPt.vi"("x"=w22, "sample length"=3) -> ("mean"=→"Rate [K/min]":dbl)  [unwired: 2 in, 1 out]
          n162 = call "Convert to Dynamic Data7"("Array"=w33) -> ("Dynamic Data Type"=w36:dynamicdata)  [unwired: 3 in]
          n163 = call "Convert to Dynamic Data8"("Array"=w31) -> ("Dynamic Data Type"=w35:dynamicdata)  [unwired: 3 in]
          n164 = case shown="False" "Measure R-T" {
            tunnel: w36 -> [_ w165]
            tunnel: w35 -> [_ w164]
            frame False {
            }
            frame True {
              n165 = call "Build XY Graph2"("Y Input"=w164, "X Input"=w165) -> ("XY Graph"=→"R-T":cluster{"X":dbl[], "Y":dbl[]}[])  [unwired: 8 in, 1 out]
              n166 = call "Time Delay16"("Delay Time (s)"="Period [s]") -> ()  [unwired: 10 in, 1 out]
            }
          }
          n167 = call "Convert to Dynamic Data9"("Array"=w33) -> ("Dynamic Data Type"=w32:dynamicdata)  [unwired: 3 in]
          n168 = call "Convert to Dynamic Data10"("Array"=w31) -> ("Dynamic Data Type"=w30:dynamicdata)  [unwired: 3 in]
          n169 = Merge Signals(w32, w30) -> (w34:dynamicdata)
          n170 = case shown="False" "Save R-T" {
            tunnel: w34 -> [_ w166]
            frame False {
            }
            frame True {
              n171 = flat-sequence {
                tunnel: w166 -> [w167]
                frame #0 {
                  n172 = call "Write To Measurement File2"("Signals"=w167, "Reset"=TRUE) -> ()  [unwired: 15 in, 3 out]
                }
                frame #1 {
                  n173 = local write "Save R-T"(FALSE) -> ()
                }
              }
            }
          }
          n174 = case shown="True" "Measure R-H" {
            frame False {
            }
            frame True {
              n175 = local write "Measure R-T"(FALSE) -> ()
            }
          }
        }
      }
      frame #1 {
        # "interlocks"
        n176 = Index Array(array="Set Temp [K]  Rate [K/min]", index (col)=0) -> (element=w416:dbl[])  [unwired: 1 in]
        n177 = Index Array(array="Set Temp [K]  Rate [K/min]", index (col)=1) -> (element=w423:dbl[])  [unwired: 1 in]
        n178 = Array Max & Min(array=w416) -> (max value=w410:dbl, min value=w419:dbl)  [unwired: 2 out]
        n179 = while {
          tunnel: "Set Temp [K]  Rate [K/min]" -> [w441]
          tunnel: w408 -> [w439]
          tunnel: w407 -> [w438]
          tunnel: w406 -> [w437]
          tunnel: w404 -> [w428]
          tunnel: w403 -> [w427]
          tunnel: w402 -> [w426]
          i -> [w440]
          stop <- w429 stop-if-true
          n180 = Matrix Size(0:w441) -> (1:w442:i32)  [unwired: 1 out]
          n181 = Less Or Equal?(x=w442, y=w440) -> (x <= y?=w432:bool)
          n182 = Index Array(array=w441, index (row)=w440) -> (element=w443:dbl[])  [unwired: 1 in]
          n183 = Index Array(array=w443, index=1) -> (element=w435:dbl)
          n184 = Index Array(array=w443, index=0) -> (element=w434:dbl)
          n185 = Multiply(x=w435, y=w434) -> (x*y=w436:dbl)
          n186 = Equal To 0?(x=w436) -> (x = 0?=w433:bool)
          n187 = Or(x=w433, y=w432) -> (x .or. y?=w431:bool)
          n188 = case shown="False" w431 {
            tunnel: w439 -> [w455 _]
            tunnel: w435 -> [w454 _]
            tunnel: w438 -> [w448 _]
            tunnel: w437 -> [w453 _]
            tunnel: w434 -> [w452 _]
            tunnel: [w451 FALSE ("Boolean")] -> w430
            tunnel: w428 -> [w449 _]
            tunnel: w427 -> [w447 _]
            tunnel: w426 -> [w446 _]
            frame False {
              n189 = stacked-sequence {
                tunnel: w455 -> [w456 w571]
                tunnel: w452 -> [w461 _]
                tunnel: w454 -> [w460 _]
                tunnel: w448 -> [w459 w570]
                tunnel: w453 -> [_ w569]
                tunnel: w452 -> [_ w568]
                tunnel: [_ w567] -> w451
                tunnel: "Field [T]" -> [w458 w566]
                tunnel: w449 -> [w457 _]
                tunnel: w447 -> [_ w565]
                tunnel: w446 -> [_ w564]
                frame #0 {
                  n190 = flat-sequence {
                    tunnel: w457 -> [w466]
                    tunnel: w461 -> [w465]
                    tunnel: w460 -> [w464]
                    tunnel: w456 -> [w462]
                    tunnel: w459 -> [w528]
                    tunnel: w458 -> [w526]
                    frame #0 {
                      n191 = case shown="False" "Temp control off" {
                        tunnel: w466 -> [w469 _]
                        tunnel: w465 -> [w472 _]
                        tunnel: w464 -> [w471 _]
                        tunnel: w462 -> [w467 _]
                        frame False {
                          n192 = case shown="False" "Main sorb T control" {
                            tunnel: w469 -> [_ w474]
                            tunnel: [w473 w474] -> w468
                            tunnel: w467 -> [w473 _]
                            frame False {
                            }
                            frame True {
                            }
                          }
                          n193 = stacked-sequence {
                            tunnel: w468 -> [w475 _ w485 _ w495 w499]
                            tunnel: w472 -> [_ _ _ _ w494 _]
                            tunnel: w471 -> [_ _ w486 _ _ _]
                            tunnel: "Main sorb T control" -> [w476 _ _ _ _ w500]
                            frame #0 {
                              n194 = case shown="False" w476 {
                                tunnel: ["OUTMODE 1, 1, 2, 1" ("write buffer") "OUTMODE1,1,1,1" ("write buffer")] -> w477
                                frame False {
                                }
                                frame True {
                                }
                              }
                              n195 = Concatenate Strings(w477, "\n") -> (w478:string)
                              n196 = VISA Write(VISA resource name=w475, write buffer=w478) -> ()  [unwired: 1 in, 3 out]
                            }
                            frame #1 {
                              n197 = Wait (ms)(milliseconds to wait=u32 50) -> ()  [unwired: 1 out]
                            }
                            frame #2 {
                              n198 = case shown="False" "T-ramp off" {
                                tunnel: ["RAMP 1, 1," ("write buffer") "RAMP 1, 0," ("write buffer")] -> w484
                                frame False {
                                }
                                frame True {
                                }
                              }
                              n199 = Number To Fractional String(number=w486) -> (F-format string=w487:string)  [unwired: 3 in]
                              n200 = Concatenate Strings(w484, w487, "\n") -> (w488:string)
                              n201 = VISA Write(VISA resource name=w485, write buffer=w488) -> ()  [unwired: 1 in, 3 out]
                            }
                            frame #3 {
                              n202 = Wait (ms)(milliseconds to wait=u32 50) -> ()  [unwired: 1 out]
                            }
                            frame #4 {
                              n203 = Number To Fractional String(number=w494) -> (F-format string=w493:string)  [unwired: 3 in]
                              n204 = Concatenate Strings("SETP 1," ("write buffer"), w493, "\n") -> (w497:string)
                              n205 = VISA Write(VISA resource name=w495, write buffer=w497) -> ()  [unwired: 1 in, 3 out]
                            }
                            frame #5 {
                              n206 = flat-sequence {
                                tunnel: w500 -> [w502]
                                tunnel: w499 -> [w501]
                                frame #0 {
                                n207 = while {
                                tunnel: w502 -> [w505]
                                tunnel: w501 -> [w504]
                                i -> [w503]
                                stop <- w517 stop-if-true
                                n208 = case shown="False" w505 {
                                tunnel: ["KRDG? B" ("write buffer") "KRDG? A" ("write buffer")] -> w506
                                frame False {
                                }
                                frame True {
                                }
                                }
                                n209 = Concatenate Strings(w506, "\n") -> (w511:string)
                                n210 = VISA Write(VISA resource name=w504, write buffer=w511) -> (VISA resource name out=w510:refnum<visa-resource-name>)  [unwired: 1 in, 2 out]
                                n211 = Multiply(x="Wait T-stable [min]", y=60) -> (x*y=w516:i32)
                                n212 = Less?(x=w516, y=w503) -> (x < y?=w515:bool)
                                n213 = VISA Read(VISA resource name=w510, byte count=u32 100) -> (read buffer=w508:string)  [unwired: 1 in, 3 out]
                                n214 = Or(x=w515, y="Skip") -> (x .or. y?=w517:bool)
                                n215 = Wait (ms)(milliseconds to wait=1000) -> ()  [unwired: 1 out]
                                n216 = Fract/Exp String To Number(string=w508) -> (number=→"temp [K]":dbl)  [unwired: 3 in, 1 out]
                                "Waiting T-stability" <- TRUE
                                }
                                }
                                frame #1 {
                                w523 = FALSE
                                n217 = local write "Skip"(w523) -> ()
                                n218 = local write "Reset"(TRUE) -> ()
                                n219 = local write "Waiting T-stability"(w523) -> ()
                                }
                              }
                            }
                          }
                        }
                        frame True {
                          n220 = local write "Reset"(TRUE) -> ()
                        }
                      }
                    }
                    frame #1 {
                      n221 = case shown="True" "Set Initial Field" {
                        tunnel: w528 -> [_ w531]
                        tunnel: w526 -> [_ w529]
                        frame False {
                        }
                        frame True {
                          n222 = stacked-sequence {
                            tunnel: w531 -> [w532 w535 _ w553 _ w558 _]
                            tunnel: 0.2 -> [_ _ _ w543 _ _ _]
                            tunnel: w529 -> [_ w533 _ _ _ _ _]
                            frame #0 {
                              n223 = VISA Clear(VISA resource name=w532) -> ()  [unwired: 1 in, 2 out]
                            }
                            frame #1 {
                              # "set set field"
                              n224 = Number To Fractional String(number=w533, width (-)=i16 6, precision (6)=i16 3) -> (F-format string=w538:string)  [unwired: 1 in]
                              n225 = Concatenate Strings("S [%][MID] " ("string"), w538) -> (w534:string)
                              n226 = Concatenate Strings(w534, "\r") -> (w537:string)
                              n227 = VISA Write(VISA resource name=w535, write buffer=w537) -> ()  [unwired: 1 in, 3 out]
                            }
                            frame #2 {
                              n228 = Wait (ms)(milliseconds to wait=500) -> ()  [unwired: 1 out]
                            }
                            frame #3 {
                              # "set rate"
                              n229 = Divide(x=w543, y=60.0) -> (x/y=w548:dbl)
                              n230 = Divide(x=w548, y=0.09797) -> (x/y=w546:dbl)
                              n231 = Number To Fractional String(number=w546, width (-)=i16 6, precision (6)=i16 3) -> (F-format string=w551:string)  [unwired: 1 in]
                              n232 = Concatenate Strings("S R " ("string"), w551) -> (w550:string)
                              n233 = Concatenate Strings(w550, "\r") -> (w555:string)
                              n234 = VISA Write(VISA resource name=w553, write buffer=w555) -> ()  [unwired: 1 in, 3 out]
                            }
                            frame #4 {
                              n235 = Wait (ms)(milliseconds to wait=500) -> ()  [unwired: 1 out]
                            }
                            frame #5 {
                              # "Go to set field"
                              n236 = Concatenate Strings("R [%][MID]" ("data"), "\r") -> (w560:string)
                              n237 = VISA Write(VISA resource name=w558, write buffer=w560) -> ()  [unwired: 1 in, 3 out]
                            }
                            frame #6 {
                              n238 = Multiply(x="Wait [min]", y=60000) -> (x*y=w563:i32)
                              n239 = Wait (ms)(milliseconds to wait=w563) -> ()  [unwired: 1 out]
                            }
                          }
                        }
                      }
                    }
                  }
                }
                frame #1 {
                  n240 = flat-sequence {
                    tunnel: [w587] -> w578
                    tunnel: [w588] -> w577
                    tunnel: ["Set Field [T]   Rate [T/min]"] -> w576
                    tunnel: w570 -> [w588]
                    tunnel: w569 -> [w587]
                    tunnel: w566 -> [w584]
                    tunnel: w578 -> [w612]
                    tunnel: [w612] -> w575
                    tunnel: [w611] -> w574
                    tunnel: w577 -> [w611]
                    tunnel: [w611] -> w573
                    tunnel: [w610] -> w572
                    tunnel: w576 -> [w610]
                    tunnel: w575 -> [w621]
                    tunnel: w574 -> [w620]
                    tunnel: w573 -> [w619]
                    tunnel: w572 -> [w618]
                    tunnel: w571 -> [w617]
                    tunnel: w568 -> [w616]
                    tunnel: [w615] -> w567
                    tunnel: w565 -> [w614]
                    tunnel: w564 -> [w613]
                    frame #0 {
                      # "interlocks"
                      n241 = Index Array(array="Set Field [T]   Rate [T/min]", index (col)=0) -> (element=w596:dbl[])  [unwired: 1 in]
                      n242 = Array Max & Min(array=w596) -> (max value=w589:dbl, min value=w599:dbl)  [unwired: 2 out]
                      n243 = Index Array(array="Set Field [T]   Rate [T/min]", index (col)=1) -> (element=w607:dbl[])  [unwired: 1 in]
                      n244 = Array Max & Min(array=w607) -> (max value=w601:dbl, min value=w604:dbl)  [unwired: 2 out]
                      n245 = Greater?(x=w589, y=10) -> (0:w590:bool)
                      n246 = Less?(x=w599, y=-10) -> (x < y?=w600:bool)
                      n247 = Greater?(x=w584, y=10) -> (0:w583:bool)
                      n248 = Less?(x=w584, y=-10) -> (x < y?=w582:bool)
                      n249 = Or(x=w590, y=w600) -> (x .or. y?=w580:bool)
                      n250 = Or(x=w583, y=w582) -> (x .or. y?=w581:bool)
                      n251 = Greater?(x=w601, y=0.6) -> (0:w606:bool)
                      n252 = Less?(x=w604, y=-0.6) -> (x < y?=w605:bool)
                      n253 = Or(x=w581, y=w580) -> (x .or. y?=w579:bool)
                      n254 = call "Display Message to User4"("Enable"=w579) -> ("OK"=w609:bool)  [unwired: 9 in, 1 out]
                      n255 = Or(x=w606, y=w605) -> (x .or. y?=w608:bool)
                      n256 = call "Display Message to User3"("Enable"=w608) -> ("OK"=w591:bool)  [unwired: 9 in, 1 out]
                      n257 = Or(x=w609, y=w591) -> (x .or. y?=w592:bool)
                      n258 = Stop(stop? (T)=w592) -> ()
                    }
                    frame #1 {
                    }
                    frame #2 {
                      n259 = while {
                        tunnel: w621 -> [w641]
                        tunnel: w620 -> [w640]
                        tunnel: w619 -> [w635]
                        tunnel: w618 -> [w632]
                        tunnel: w617 -> [w631]
                        tunnel: w616 -> [w630]
                        tunnel: [w624] -> w615
                        tunnel: w614 -> [w623]
                        tunnel: w613 -> [w622]
                        i -> [w636]
                        stop <- w625 stop-if-true
                        n260 = Matrix Size(0:w632) -> (1:w633:i32)  [unwired: 1 out]
                        n261 = Less Or Equal?(x=w633, y=w636) -> (x <= y?=w627:bool)
                        n262 = Index Array(array=w632, index (row)=w636) -> (element=w637:dbl[])  [unwired: 1 in]
                        n263 = Index Array(array=w637, index=1) -> (element=w629:dbl)
                        n264 = Equal To 0?(x=w629) -> (x = 0?=w628:bool)
                        n265 = Or(x=w628, y=w627) -> (x .or. y?=w626:bool)
                        n266 = Index Array(array=w637, index=0) -> (element=w634:dbl)
                        n267 = case shown="False" w626 {
                          tunnel: w641 -> [w651 _]
                          tunnel: w640 -> [w650 _]
                          tunnel: w629 -> [w649 _]
                          tunnel: w635 -> [w648 _]
                          tunnel: w634 -> [w647 _]
                          tunnel: w631 -> [w646 _]
                          tunnel: w630 -> [w645 _]
                          tunnel: [w644 FALSE] -> w624
                          tunnel: w623 -> [w643 _]
                          tunnel: w622 -> [w642 _]
                          frame False {
                            n268 = stacked-sequence {
                              tunnel: w651 -> [_ w737]
                              tunnel: w650 -> [_ w736]
                              tunnel: w648 -> [w654 _]
                              tunnel: w647 -> [w653 w735]
                              tunnel: w649 -> [w652 _]
                              tunnel: w646 -> [_ w734]
                              tunnel: w645 -> [_ w733]
                              tunnel: [_ w732] -> w644
                              tunnel: w643 -> [_ w731]
                              tunnel: w642 -> [_ w730]
                              frame #0 {
                                n269 = stacked-sequence {
                                tunnel: w653 -> [_ _ w662 _ w705 _ _ _ _ _]
                                tunnel: w654 -> [w655 _ w658 _ w702 _ w721 _ w726 _]
                                tunnel: w652 -> [_ _ _ _ _ _ w714 _ _ _]
                                frame #0 {
                                n270 = VISA Clear(VISA resource name=w655) -> ()  [unwired: 1 in, 2 out]
                                }
                                frame #1 {
                                n271 = Wait (ms)(milliseconds to wait=500) -> ()  [unwired: 1 out]
                                }
                                frame #2 {
                                # "Read Magnetic Field"
                                # "for safety"
                                # "polarity"
                                n272 = stacked-sequence {
                                seq-local: [w663 _ _ _ _ _ _ _] -> [_ w666 _ _ _ _ _ _]
                                seq-local: [_ w664 _ _ _ _ _ _] -> [_ _ w668 _ _ _ _ _]
                                seq-local: [_ w665 _ _ _ _ _ _] -> [_ _ w667 _ _ _ _ _]
                                seq-local: [_ _ w668 _ _ _ _ _] -> [_ _ _ w671 _ _ _ _]
                                seq-local: [_ _ w667 _ _ _ _ _] -> [_ _ _ w670 _ _ _ _]
                                seq-local: [_ _ _ w673 _ _ _ _] -> [_ _ _ _ w676 _ _ _]
                                seq-local: [_ _ _ w672 _ _ _ _] -> [_ _ _ _ w677 _ _ _]
                                seq-local: [_ _ _ _ w676 _ _ _] -> [_ _ _ _ _ w688 _ _]
                                seq-local: [_ _ _ _ w677 _ _ _] -> [_ _ _ _ _ w686 _ _]
                                seq-local: [_ _ _ _ _ w687 _ _] -> [_ _ _ _ _ _ _ w691]
                                seq-local: [_ _ _ _ _ w685 _ _] -> [_ _ _ _ _ _ _ w690]
                                tunnel: w658 -> [w663 _ _ _ _ _ _ _]
                                tunnel: [_ _ _ _ _ w678 _ _] -> w659
                                frame #0 {
                                }
                                frame #1 {
                                n273 = VISA Clear(VISA resource name=w666) -> (VISA resource name out=w664:refnum<visa-resource-name>, error out=w665:errorcluster)  [unwired: 1 in]
                                }
                                frame #2 {
                                n274 = call "Time Delay4"() -> ()  [unwired: 11 in, 1 out]
                                }
                                frame #3 {
                                n275 = Concatenate Strings("G O" ("Command"), "\r") -> (w674:string)
                                n276 = VISA Write(VISA resource name=w671, write buffer=w674, error in (no error)=w670) -> (VISA resource name out=w673:refnum<visa-resource-name>, error out=w672:errorcluster)  [unwired: 1 out]
                                }
                                frame #4 {
                                n277 = call "Time Delay5"() -> ()  [unwired: 11 in, 1 out]
                                }
                                frame #5 {
                                n278 = VISA Read(VISA resource name=w688, byte count=u32 30, error in (no error)=w686) -> (VISA resource name out=w687:refnum<visa-resource-name>, read buffer=w682:string, error out=w685:errorcluster)  [unwired: 1 out]
                                n279 = Match Pattern(string=w682, regular expression="OUTPUT:") -> (after substring=w680:string)  [unwired: 1 in, 3 out]
                                n280 = Match Pattern(string=w680, regular expression=" TESLA") -> (before substring=w679:string)  [unwired: 1 in, 3 out]
                                n281 = Fract/Exp String To Number(string=w679, offset=0) -> (number=w678:dbl)  [unwired: 2 in, 1 out]
                                }
                                frame #6 {
                                n282 = call "Time Delay13"() -> ()  [unwired: 11 in, 1 out]
                                }
                                frame #7 {
                                n283 = VISA Close(VISA resource name=w691, error in (no error)=w690) -> ()  [unwired: 1 out]
                                }
                                }
                                n284 = Absolute Value(x=w659) -> (abs(x)=w660:dbl)
                                n285 = Less?(x=w660, y=0.01) -> (x < y?=w657:bool)
                                n286 = case shown="False" w657 {
                                tunnel: w662 -> [_ w693]
                                tunnel: w658 -> [_ w694]
                                frame False {
                                }
                                frame True {
                                n287 = Greater Or Equal To 0?(x=w693) -> (x >= 0?=w692:bool)
                                n288 = case shown="True" w692 {
                                tunnel: ["D [-]" ("data") "D [+]" ("data")] -> w695
                                frame False {
                                }
                                frame True {
                                }
                                }
                                n289 = Concatenate Strings(w695, "\r") -> (w697:string)
                                n290 = VISA Write(VISA resource name=w694, write buffer=w697) -> ()  [unwired: 1 in, 3 out]
                                }
                                }
                                }
                                frame #3 {
                                n291 = Wait (ms)(milliseconds to wait=500) -> ()  [unwired: 1 out]
                                }
                                frame #4 {
                                # "set set field"
                                n292 = Number To Fractional String(number=w705, width (-)=i16 6, precision (6)=i16 3) -> (F-format string=w706:string)  [unwired: 1 in]
                                n293 = Concatenate Strings("S [%][MID] " ("string"), w706) -> (w701:string)
                                n294 = Concatenate Strings(w701, "\r") -> (w704:string)
                                n295 = VISA Write(VISA resource name=w702, write buffer=w704) -> ()  [unwired: 1 in, 3 out]
                                }
                                frame #5 {
                                n296 = Wait (ms)(milliseconds to wait=500) -> ()  [unwired: 1 out]
                                }
                                frame #6 {
                                # "set rate"
                                n297 = Divide(x=w714, y=60.0) -> (x/y=w716:dbl)
                                n298 = Divide(x=w716, y=0.09797) -> (x/y=w711:dbl)
                                n299 = Number To Fractional String(number=w711, width (-)=i16 6, precision (6)=i16 3) -> (F-format string=w719:string)  [unwired: 1 in]
                                n300 = Concatenate Strings("S R " ("string"), w719) -> (w718:string)
                                n301 = Concatenate Strings(w718, "\r") -> (w723:string)
                                n302 = VISA Write(VISA resource name=w721, write buffer=w723) -> ()  [unwired: 1 in, 3 out]
                                }
                                frame #7 {
                                n303 = Wait (ms)(milliseconds to wait=500) -> ()  [unwired: 1 out]
                                }
                                frame #8 {
                                # "Go to set field"
                                n304 = Concatenate Strings("R [%][MID]" ("data"), "\r") -> (w728:string)
                                n305 = VISA Write(VISA resource name=w726, write buffer=w728) -> ()  [unwired: 1 in, 3 out]
                                }
                                frame #9 {
                                n306 = Wait (ms)(milliseconds to wait=500) -> ()  [unwired: 1 out]
                                }
                                }
                              }
                              frame #1 {
                                n307 = while {
                                tunnel: w737 -> [w759]
                                tunnel: w736 -> [w760]
                                tunnel: w735 -> [w758]
                                tunnel: w734 -> [w756]
                                tunnel: w733 -> [w755]
                                shift-right: [w747] -> _
                                shift-left: _ -> [w754]
                                shift-right: [w750] -> _
                                shift-left: _ -> [w753]
                                shift-right: [w749] -> _
                                shift-left: _ -> [w752]
                                shift-right: [w748] -> _
                                shift-left: _ -> [w751]
                                tunnel: ["Stop"] -> w732
                                tunnel: w731 -> [w743]
                                tunnel: w730 -> [w742]
                                shift-right: [w741] -> _
                                shift-left: _ -> [w740]
                                shift-right: [w739] -> _
                                shift-left: _ -> [w738]
                                stop <- w746 stop-if-true
                                n308 = stacked-sequence {
                                seq-local: [w767 _ _ _ _ _] -> [_ w832 _ _ _ _]
                                seq-local: [w766 _ _ _ _ _] -> [_ w831 _ _ _ _]
                                seq-local: [_ w833 _ _ _ _] -> [_ _ w853 _ _ _]
                                seq-local: [_ w823 _ _ _ _] -> [_ _ w852 _ _ _]
                                seq-local: [_ w831 _ _ _ _] -> [_ _ w844 _ _ _]
                                seq-local: [_ w822 _ _ _ _] -> [_ _ w842 _ _ _]
                                seq-local: [_ _ w853 _ _ _] -> [_ _ _ w896 _ _]
                                seq-local: [_ _ w852 _ _ _] -> [_ _ _ w895 _ _]
                                seq-local: [_ _ w843 _ _ _] -> [_ _ _ w894 _ _]
                                seq-local: [_ _ w842 _ _ _] -> [_ _ _ w887 _ _]
                                seq-local: [_ _ _ w896 _ _] -> [_ _ _ _ w961 _]
                                seq-local: [_ _ _ w895 _ _] -> [_ _ _ _ w954 _]
                                seq-local: [_ _ _ w894 _ _] -> [_ _ _ _ w955 _]
                                seq-local: [_ _ _ w894 _ _] -> [_ _ _ _ _ _]
                                seq-local: [_ _ _ w886 _ _] -> [_ _ _ _ w951 _]
                                seq-local: [w763 _ _ _ _ _] -> [_ _ _ _ w898 _]
                                seq-local: [w762 _ _ _ _ _] -> [_ _ _ _ w897 _]
                                tunnel: w759 -> [w768 _ _ _ _ _]
                                tunnel: w760 -> [w766 _ _ _ _ _]
                                tunnel: w756 -> [_ w824 _ _ _ _]
                                tunnel: w758 -> [_ _ w851 _ _ _]
                                tunnel: [_ _ w849 _ _ _] -> w757
                                tunnel: [_ _ _ _ w961 _] -> _
                                tunnel: w755 -> [_ _ _ _ w957 _]
                                tunnel: [_ _ _ _ w938 _] -> w747
                                tunnel: w754 -> [_ _ _ _ w950 _]
                                tunnel: [_ _ _ _ w932 _] -> w750
                                tunnel: w753 -> [_ _ _ _ w945 _]
                                tunnel: [_ _ _ _ w934 _] -> w749
                                tunnel: w752 -> [_ _ _ _ w904 _]
                                tunnel: [_ _ _ _ w935 _] -> w748
                                tunnel: w751 -> [_ _ _ _ w953 _]
                                tunnel: w743 -> [w765 w820 _ _ w899 _]
                                tunnel: w742 -> [w764 _ _ _ _ _]
                                tunnel: [_ _ _ _ w909 _] -> w741
                                tunnel: w740 -> [_ _ _ _ w903 _]
                                tunnel: [_ _ _ _ w907 _] -> w739
                                tunnel: w738 -> [_ _ _ _ w902 _]
                                frame #0 {
                                n309 = case shown="False" w765 {
                                tunnel: w768 -> [w773 w818]
                                tunnel: [w773 w817] -> w767
                                tunnel: w764 -> [w769 _]
                                tunnel: [w772 w816] -> w763
                                tunnel: [w771 w816] -> w762
                                frame False {
                                n310 = flat-sequence {
                                tunnel: [w778] -> w772
                                tunnel: w769 -> [w777]
                                tunnel: [w776] -> w770
                                tunnel: [w799] -> w771
                                tunnel: w770 -> [w798]
                                frame #0 {
                                n311 = flat-sequence {
                                tunnel: w777 -> [w782]
                                tunnel: [w781] -> w775
                                tunnel: w775 -> [w784]
                                tunnel: [w784] -> w774
                                tunnel: [w785] -> w780
                                tunnel: w774 -> [w787]
                                tunnel: [w788] -> w779
                                tunnel: w780 -> [w788]
                                tunnel: w779 -> [w793]
                                tunnel: [w791] -> w778
                                tunnel: [w790] -> w776
                                frame #0 {
                                n312 = VISA Clear(VISA resource name=w782) -> (VISA resource name out=w781:refnum<visa-resource-name>)  [unwired: 1 in, 1 out]
                                }
                                frame #1 {
                                n313 = Wait (ms)(milliseconds to wait=5) -> ()  [unwired: 1 out]
                                }
                                frame #2 {
                                n314 = VISA Write(VISA resource name=w787, write buffer="OUTP? 1" ("write buffer 2")) -> (VISA resource name out=w785:refnum<visa-resource-name>)  [unwired: 1 in, 2 out]
                                }
                                frame #3 {
                                n315 = Wait (ms)(milliseconds to wait=5) -> ()  [unwired: 1 out]
                                }
                                frame #4 {
                                n316 = VISA Read(VISA resource name=w793, byte count=u32 360) -> (VISA resource name out=w790:refnum<visa-resource-name>, read buffer=w792:string)  [unwired: 1 in, 2 out]
                                n317 = Fract/Exp String To Number(string=w792, offset=0) -> (number=w791:dbl)  [unwired: 3 out]
                                "Lockin x (V)" <- w791
                                }
                                }
                                }
                                frame #1 {
                                n318 = flat-sequence {
                                tunnel: w798 -> [w803]
                                tunnel: [w802] -> w797
                                tunnel: w797 -> [w805]
                                tunnel: [w805] -> w796
                                tunnel: [w806] -> w801
                                tunnel: w796 -> [w808]
                                tunnel: [w809] -> w800
                                tunnel: w801 -> [w809]
                                tunnel: w800 -> [w813]
                                tunnel: [w811] -> w799
                                frame #0 {
                                n319 = VISA Clear(VISA resource name=w803) -> (VISA resource name out=w802:refnum<visa-resource-name>)  [unwired: 1 in, 1 out]
                                }
                                frame #1 {
                                n320 = Wait (ms)(milliseconds to wait=5) -> ()  [unwired: 1 out]
                                }
                                frame #2 {
                                n321 = VISA Write(VISA resource name=w808, write buffer="OUTP? 2" ("write buffer 2")) -> (VISA resource name out=w806:refnum<visa-resource-name>)  [unwired: 1 in, 2 out]
                                }
                                frame #3 {
                                n322 = Wait (ms)(milliseconds to wait=5) -> ()  [unwired: 1 out]
                                }
                                frame #4 {
                                n323 = VISA Read(VISA resource name=w813, byte count=u32 360) -> (read buffer=w812:string)  [unwired: 1 in, 3 out]
                                n324 = Fract/Exp String To Number(string=w812, offset=0) -> (number=w811:dbl)  [unwired: 3 out]
                                "Lockin y (V)" <- w811
                                }
                                }
                                }
                                }
                                }
                                frame True {
                                w816 = 0.0
                                n325 = VISA Write(VISA resource name=w818, write buffer="SENS:DATA:LATest?") -> (VISA resource name out=w817:refnum<visa-resource-name>)  [unwired: 1 in, 2 out]
                                }
                                }
                                }
                                frame #1 {
                                n326 = Concatenate Strings("KRDG? A" ("write buffer"), "\n") -> (w829:string)
                                n327 = VISA Write(VISA resource name=w824, write buffer=w829) -> (VISA resource name out=w827:refnum<visa-resource-name>)  [unwired: 1 in, 2 out]
                                n328 = VISA Read(VISA resource name=w827, byte count=u32 100) -> (VISA resource name out=w822:refnum<visa-resource-name>, read buffer=w825:string)  [unwired: 1 in, 2 out]
                                n329 = case shown="True" w820 {
                                tunnel: [w835 w841] -> w833
                                tunnel: w832 -> [w835 w837]
                                tunnel: [0.0 w836] -> w823
                                frame False {
                                }
                                frame True {
                                n330 = VISA Read(VISA resource name=w837, byte count=u32 360) -> (VISA resource name out=w841:refnum<visa-resource-name>, read buffer=w839:string)  [unwired: 1 in, 2 out]
                                n331 = Fract/Exp String To Number(string=w839, offset=0) -> (number=w836:dbl)  [unwired: 3 out]
                                }
                                }
                                "Delta reading [Ohm]" <- w823
                                n332 = Fract/Exp String To Number(string=w825) -> (number=→"VTI [K]":dbl)  [unwired: 3 in, 1 out]
                                }
                                frame #2 {
                                # "Read Magnetic Field"
                                n333 = stacked-sequence {
                                seq-local: [w854 _ _ _ _ _ _ _] -> [_ w857 _ _ _ _ _ _]
                                seq-local: [_ w855 _ _ _ _ _ _] -> [_ _ w859 _ _ _ _ _]
                                seq-local: [_ w856 _ _ _ _ _ _] -> [_ _ w858 _ _ _ _ _]
                                seq-local: [_ _ w859 _ _ _ _ _] -> [_ _ _ w862 _ _ _ _]
                                seq-local: [_ _ w858 _ _ _ _ _] -> [_ _ _ w861 _ _ _ _]
                                seq-local: [_ _ _ w864 _ _ _ _] -> [_ _ _ _ w867 _ _ _]
                                seq-local: [_ _ _ w863 _ _ _ _] -> [_ _ _ _ w868 _ _ _]
                                seq-local: [_ _ _ _ w867 _ _ _] -> [_ _ _ _ _ w879 _ _]
                                seq-local: [_ _ _ _ w868 _ _ _] -> [_ _ _ _ _ w877 _ _]
                                seq-local: [_ _ _ _ _ w878 _ _] -> [_ _ _ _ _ _ _ w883]
                                seq-local: [_ _ _ _ _ w876 _ _] -> [_ _ _ _ _ _ _ w882]
                                tunnel: w844 -> [w854 _ _ _ _ _ _ _]
                                tunnel: [_ _ _ _ _ w869 _ _] -> w843
                                frame #0 {
                                }
                                frame #1 {
                                n334 = VISA Clear(VISA resource name=w857) -> (VISA resource name out=w855:refnum<visa-resource-name>, error out=w856:errorcluster)  [unwired: 1 in]
                                }
                                frame #2 {
                                n335 = call "Time Delay2"() -> ()  [unwired: 11 in, 1 out]
                                }
                                frame #3 {
                                n336 = Concatenate Strings("G O" ("Command"), "\r") -> (w865:string)
                                n337 = VISA Write(VISA resource name=w862, write buffer=w865, error in (no error)=w861) -> (VISA resource name out=w864:refnum<visa-resource-name>, error out=w863:errorcluster)  [unwired: 1 out]
                                }
                                frame #4 {
                                n338 = call "Time Delay3"() -> ()  [unwired: 11 in, 1 out]
                                }
                                frame #5 {
                                n339 = VISA Read(VISA resource name=w879, byte count=u32 30, error in (no error)=w877) -> (VISA resource name out=w878:refnum<visa-resource-name>, read buffer=w873:string, error out=w876:errorcluster)  [unwired: 1 out]
                                n340 = Match Pattern(string=w873, regular expression="OUTPUT:") -> (after substring=w871:string)  [unwired: 1 in, 3 out]
                                n341 = Match Pattern(string=w871, regular expression=" TESLA") -> (before substring=w870:string)  [unwired: 1 in, 3 out]
                                n342 = Fract/Exp String To Number(string=w870, offset=0) -> (number=w869:dbl)  [unwired: 2 in, 1 out]
                                }
                                frame #6 {
                                n343 = call "Time Delay12"() -> ()  [unwired: 11 in, 1 out]
                                }
                                frame #7 {
                                n344 = VISA Close(VISA resource name=w883, error in (no error)=w882) -> (error out=→"error out 3":errorcluster)
                                }
                                }
                                "Magnetic Field [T]" <- w843
                                n345 = Equal To 0?(x=w843) -> (x = 0?=w846:bool)
                                n346 = case shown="False" w846 {
                                tunnel: w843 -> [w884 _]
                                tunnel: [w884 1.1] -> w845
                                frame False {
                                }
                                frame True {
                                }
                                }
                                n347 = Subtract(x=w845, y=w851) -> (x-y=w847:dbl)
                                n348 = Absolute Value(x=w847) -> (abs(x)=w848:dbl)
                                n349 = Less?(x=w848, y=0.03) -> (x < y?=w849:bool)
                                }
                                frame #3 {
                                n350 = Concatenate Strings("KRDG? B" ("write buffer"), "\n") -> (w892:string)
                                n351 = VISA Write(VISA resource name=w887, write buffer=w892) -> (VISA resource name out=w890:refnum<visa-resource-name>)  [unwired: 1 in, 2 out]
                                n352 = VISA Read(VISA resource name=w890, byte count=u32 100) -> (read buffer=w888:string)  [unwired: 1 in, 3 out]
                                n353 = Fract/Exp String To Number(string=w888) -> (number=w886:dbl)  [unwired: 3 in, 1 out]
                                "Sample Temp [K]" <- w886
                                }
                                frame #4 {
                                # "Y(ohm)"
                                # "X(Ohm)"
                                # "Temp"
                                # "Delta"
                                # "Field"
                                # "Time"
                                n354 = case shown="False" w899 {
                                tunnel: [w973 w974] -> w905
                                tunnel: w904 -> [_ w974]
                                tunnel: w902 -> [w973 _]
                                frame False {
                                }
                                frame True {
                                }
                                }
                                n355 = call "Convert to Dynamic Data5"("Array"=w945) -> ("Dynamic Data Type"=w930:dynamicdata)  [unwired: 3 in]
                                n356 = call "Convert to Dynamic Data6"("Array"=w905) -> ("Dynamic Data Type"=w929:dynamicdata)  [unwired: 3 in]
                                n357 = Number To Fractional String(number=w957, precision (6)=2) -> (F-format string=w958:string)  [unwired: 2 in]
                                n358 = call "Build XY Graph"("Y Input"=w929, "X Input"=w930) -> ("XY Graph"=→"R-H":cluster{"X":dbl[], "Y":dbl[]}[])  [unwired: 8 in, 1 out]
                                n359 = Format Date/Time String(time format string (%c)="%H:%M:%S%3u") -> (date/time string=w912:string)  [unwired: 2 in]
                                n360 = Fract/Exp String To Number(string=w912) -> (number=w913:dbl)  [unwired: 3 in, 1 out]
                                n361 = Path To String(path="Folder") -> (string=w941:string)
                                n362 = Match Pattern(string=w912, regular expression=":") -> (after substring=w918:string)  [unwired: 1 in, 3 out]
                                n363 = Fract/Exp String To Number(string=w918) -> (number=w920:dbl)  [unwired: 3 in, 1 out]
                                n364 = Match Pattern(string=w918, regular expression=":") -> (after substring=w914:string)  [unwired: 1 in, 3 out]
                                n365 = Multiply(x=w913, y=3600.0) -> (x*y=w917:dbl)
                                n366 = Concatenate Strings(w941, "\\", "File name", "_" ("string"), w958, "K") -> (w956:string)
                                n367 = Fract/Exp String To Number(string=w914) -> (number=w911:dbl)  [unwired: 3 in, 1 out]
                                n368 = Multiply(x=w920, y=60.0) -> (x*y=w916:dbl)
                                n369 = Build Array (concatenate)(w945, w955) -> (w931:dbl[])
                                n370 = Build Array (concatenate)(w904, w954) -> (w933:dbl[])
                                n371 = Build Array (concatenate)(w953, w951) -> (w936:dbl[])
                                n372 = Add(x=w917, y=w916) -> (x+y=w915:dbl)
                                n373 = Add(x=w915, y=w911) -> (x+y=w910:dbl)
                                n374 = Build Array (concatenate)(w950, w910) -> (w937:dbl[])
                                n375 = String To Path(string=w956) -> (path=w940:path)
                                n376 = call "Convert to Dynamic Data"("Array"=w937) -> ("Dynamic Data Type"=w946:dynamicdata)  [unwired: 3 in]
                                n377 = call "Convert to Dynamic Data2"("Array"=w931) -> ("Dynamic Data Type"=w949:dynamicdata)  [unwired: 3 in]
                                n378 = call "Convert to Dynamic Data4"("Array"=w936) -> ("Dynamic Data Type"=w947:dynamicdata)  [unwired: 3 in]
                                n379 = call "Convert to Dynamic Data3"("Array"=w933) -> ("Dynamic Data Type"=w948:dynamicdata)  [unwired: 3 in]
                                n380 = call "Convert to Dynamic Data11"("Array"=w902) -> ("Dynamic Data Type"=w901:dynamicdata)  [unwired: 3 in]
                                n381 = call "Convert to Dynamic Data12"("Array"=w903) -> ("Dynamic Data Type"=w900:dynamicdata)  [unwired: 3 in]
                                n382 = case shown="False" w899 {
                                tunnel: [w962 w972] -> w952
                                tunnel: w949 -> [w965 w971]
                                tunnel: w948 -> [_ w970]
                                tunnel: w947 -> [w966 w969]
                                tunnel: w946 -> [w967 w968]
                                tunnel: w901 -> [w964 _]
                                tunnel: w900 -> [w963 _]
                                frame False {
                                n383 = Merge Signals(w965, w963, w964, w966, w967) -> (w962:dynamicdata)
                                }
                                frame True {
                                n384 = Merge Signals(w971, w970, w969, w968) -> (w972:dynamicdata)
                                }
                                }
                                n385 = call "Write To Measurement File"("Signals"=w952, "Reset"=TRUE, "Filename"=w940) -> ("Filename Out"=→"Filename Out":path)  [unwired: 14 in, 2 out]
                                n386 = case shown="False" "Reset" {
                                tunnel: [w980 dbl[] []] -> w938
                                tunnel: w937 -> [w980 _]
                                tunnel: w936 -> [w979 _]
                                tunnel: [w979 dbl[] []] -> w935
                                tunnel: [w978 dbl[] []] -> w934
                                tunnel: w933 -> [w978 _]
                                tunnel: [w977 dbl[] []] -> w932
                                tunnel: w931 -> [w977 _]
                                tunnel: w903 -> [w976 _]
                                tunnel: [w975 dbl[] []] -> w906
                                tunnel: [w976 dbl[] []] -> w908
                                tunnel: w902 -> [w975 _]
                                frame False {
                                }
                                frame True {
                                }
                                }
                                n387 = Build Array (concatenate)(w908, w897) -> (w909:dbl[])
                                n388 = Build Array (concatenate)(w906, w898) -> (w907:dbl[])
                                }
                                frame #5 {
                                n389 = local write "Reset"(FALSE) -> ()
                                }
                                }
                                n390 = while {
                                stop <- "stop 2" continue-if-true
                                }
                                n391 = call "Time Delay"("Delay Time (s)"="period (s)") -> ()  [unwired: 1 in, 10 out]
                                n392 = case shown="True" w757 {
                                tunnel: [FALSE w989] -> w745
                                frame False {
                                }
                                frame True {
                                n393 = flat-sequence {
                                tunnel: [TRUE] -> w989
                                frame #0 {
                                n394 = Multiply(x="Wait field stable [sec]", y=1000.0) -> (x*y=w990:dbl)
                                n395 = Wait (ms)(milliseconds to wait=w990) -> ()  [unwired: 1 out]
                                }
                                frame #1 {
                                }
                                }
                                }
                                }
                                n396 = Or(x="Stop", y=w745) -> (x .or. y?=w746:bool)
                                }
                              }
                            }
                          }
                          frame True {
                          }
                        }
                        n397 = Or(x=w626, y=w624) -> (x .or. y?=w625:bool)
                      }
                    }
                  }
                }
              }
            }
            frame True {
            }
          }
          n398 = Or(x=w431, y=w430) -> (x .or. y?=w429:bool)
        }
        n399 = Array Max & Min(array=w423) -> (max value=w421:dbl)  [unwired: 3 out]
        n400 = Less?(x=w419, y=0) -> (x < y?=w420:bool)
        n401 = Greater?(x=w410, y=300) -> (0:w411:bool)
        n402 = Or(x=w411, y=w420) -> (x .or. y?=w424:bool)
        n403 = Greater?(x=w421, y=100) -> (0:w405:bool)
        n404 = call "Display Message to User2"("Enable"=w424) -> ("OK"=w425:bool)  [unwired: 9 in, 1 out]
        n405 = call "Display Message to User"("Enable"=w405) -> ("OK"=w412:bool)  [unwired: 9 in, 1 out]
        n406 = Or(x=w425, y=w412) -> (x .or. y?=w413:bool)
        n407 = Stop(stop? (T)=w413) -> ()
      }
      frame #2 {
        n408 = stacked-sequence {
          tunnel: w999 -> [w1000 w1003 _ w1021 _ w1026 _]
          tunnel: 0.1 -> [_ _ _ w1011 _ _ _]
          tunnel: 0.0 -> [_ w1001 _ _ _ _ _]
          frame #0 {
            n409 = VISA Clear(VISA resource name=w1000) -> ()  [unwired: 1 in, 2 out]
          }
          frame #1 {
            # "set set field"
            n410 = Number To Fractional String(number=w1001, width (-)=i16 6, precision (6)=i16 3) -> (F-format string=w1006:string)  [unwired: 1 in]
            n411 = Concatenate Strings("S [%][MID] " ("string"), w1006) -> (w1002:string)
            n412 = Concatenate Strings(w1002, "\r") -> (w1005:string)
            n413 = VISA Write(VISA resource name=w1003, write buffer=w1005) -> ()  [unwired: 1 in, 3 out]
          }
          frame #2 {
            n414 = Wait (ms)(milliseconds to wait=500) -> ()  [unwired: 1 out]
          }
          frame #3 {
            # "set rate"
            n415 = Divide(x=w1011, y=60.0) -> (x/y=w1016:dbl)
            n416 = Divide(x=w1016, y=0.09797) -> (x/y=w1014:dbl)
            n417 = Number To Fractional String(number=w1014, width (-)=i16 6, precision (6)=i16 3) -> (F-format string=w1019:string)  [unwired: 1 in]
            n418 = Concatenate Strings("S R " ("string"), w1019) -> (w1018:string)
            n419 = Concatenate Strings(w1018, "\r") -> (w1023:string)
            n420 = VISA Write(VISA resource name=w1021, write buffer=w1023) -> ()  [unwired: 1 in, 3 out]
          }
          frame #4 {
            n421 = Wait (ms)(milliseconds to wait=500) -> ()  [unwired: 1 out]
          }
          frame #5 {
            # "Go to set field"
            n422 = Concatenate Strings("R [%][MID]" ("data"), "\r") -> (w1028:string)
            n423 = VISA Write(VISA resource name=w1026, write buffer=w1028) -> ()  [unwired: 1 in, 3 out]
          }
          frame #6 {
            w1029 = FALSE
            n424 = local write "Measure R-H"(w1029) -> ()
            n425 = local write "Stop"(w1029) -> ()
            n426 = Wait (ms)(milliseconds to wait=500) -> ()  [unwired: 1 out]
          }
        }
      }
    }
  }
